vi "Unarchive.vi"(8 "error in":errorcluster, 11 "Path":path) -> (0 "error out":errorcluster, 1 "Archive Data.Data Files.afm":path, 2 "Archive Data.Data Files.svg":path, 3 "Archivist out":refnum<class "Archivist.lvclass">)   [LabVIEW 2019, in "Archivist.lvclass"]
uses:
  Archivist.lvclass
  Archivist.lvclass/Archivist.ctl
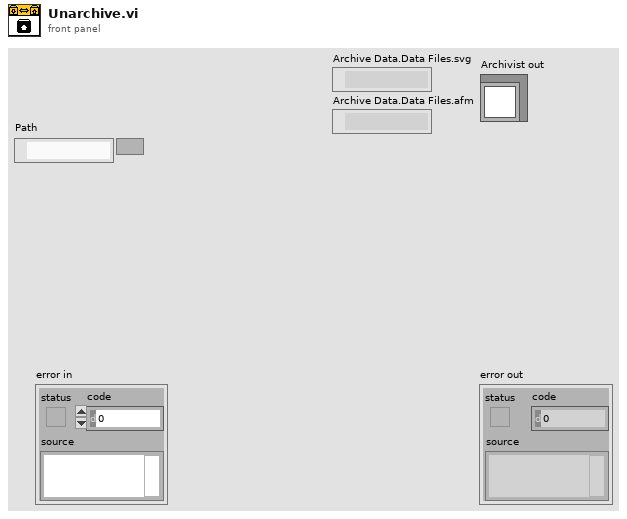
[diagram p1: front panel]
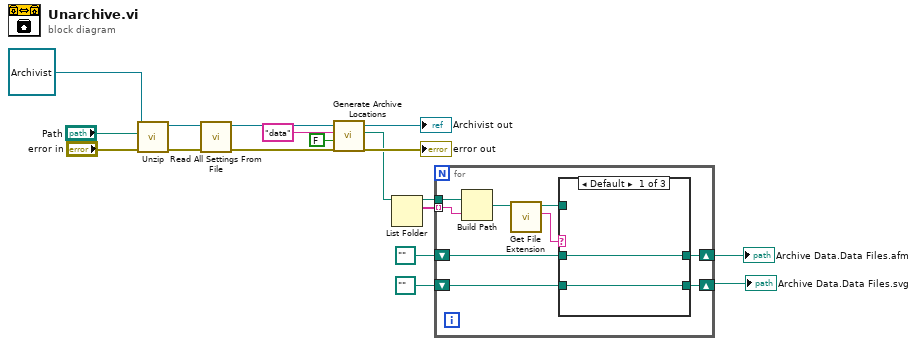
[diagram p0: block diagram]
diagram:
  n1 = call "Unzip.vi"("error in"="error in", "Path"="Path", "Archivist in"=refnum<class "Archivist.lvclass"> refnum) -> ("error out"=w16:errorcluster, "Archivist out"=w17:refnum<class "Archivist.lvclass">)  [unwired: 7 in]
  n2 = call "Read All Settings From File.vi"("error in"=w16, "Archivist in"=w17) -> ("error out"=→"error out":errorcluster, "Archivist out"=w11:refnum<class "Archivist.lvclass">)  [unwired: 8 in]
  n3 = call "Generate Archive Locations.vi"("Archive?"=FALSE, "Key"="data", "Archivist In"=w11) -> ("Path Out"=w7:path, "Archivist Out"=→"Archivist out":refnum<class "Archivist.lvclass">)  [unwired: 7 in]
  n4 = List Folder(path=w7) -> (path out=w5:path, filenames=w6:string[])  [unwired: 3 in, 2 out]
  n5 = for {
    tunnel: w6 -> [w25] mode=indexing
    tunnel: w5 -> [w26]
    shift-right: [w20] -> w2
    shift-left: path "" -> [w22]
    shift-right: [w18] -> w1
    shift-left: path "" -> [w19]
    n6 = Build Path(base path=w26, name or relative path=w25) -> (appended path=w24:path)
    n7 = call <vilib>:"Get File Extension.vi"("file"=w24) -> ("lowercase file extension"=w23:string, "dup file"=w21:path)  [unwired: 6 in, 3 out]
    n8 = case shown="Default" w23 {
      tunnel: w22 -> [w28 w30 _]
      tunnel: w21 -> [_ w29 w32]
      tunnel: [w28 w30 w32] -> w20
      tunnel: w19 -> [w27 _ w31]
      tunnel: [w27 w29 w31] -> w18
      frame Default {
      }
      frame "svg" {
      }
      frame "ibw" {
      }
    }
  }
  "Archive Data.Data Files.svg" <- w1
  "Archive Data.Data Files.afm" <- w2
